vi "PassObserverSkill.vi"(8 "error in (no error)":errorcluster, 9 "Game in":refnum<class "Game.lvclass">, 10 "Robot":refnum<class "Robot.lvclass">, 11 "PassObserverSkill in":refnum<class "PassObserverSkill.lvclass">) -> (0 "error out":errorcluster, 1 "Boolean":bool, 2 "Robot":refnum<class "Robot.lvclass">, 3 "PassObserverSkill out":refnum<class "PassObserverSkill.lvclass">)   [LabVIEW 2018, in "PassObserverSkill.lvclass"]
uses:
  PassObserverSkill.lvclass
  Robot_class/Robot.lvclass
  Game_class/Game.lvclass
  Utilities_class/Utilities.lvclass
  Robot_class/roles.ctl
  Robot_class/tactics.ctl
  Object_class/Object.lvclass/Object.ctl
  Game_class/Game.lvclass/Game.ctl
  Team_class/Team.lvclass/Team.ctl
  Parameters_class/Parameters.lvclass/Parameters.ctl
  Robot_class/Robot.lvclass/Robot.ctl
  Game_class/Read OffensiveTeam.vi
  Game_class/Read FieldRef.vi
  Game_class/Read BallRef.vi
  Game_class/Read Parameters.lvclass.vi
  Parameters_class/Read AttakingOurselves.vi
  Object_class/Read x.vi
  Object_class/Read y.vi
  Team_class/Read RobotRef.vi
  Robot_class/Read tactic.vi
  Robot_class/Write dest_x.vi
  Robot_class/Write dest_y.vi
  Robot_class/Write dest_orientation.vi
  Ball_class/Ball.lvclass
  Ally_class/Ally.lvclass
  Field_class/Field.lvclass
  Parameters_class/Parameters.lvclass
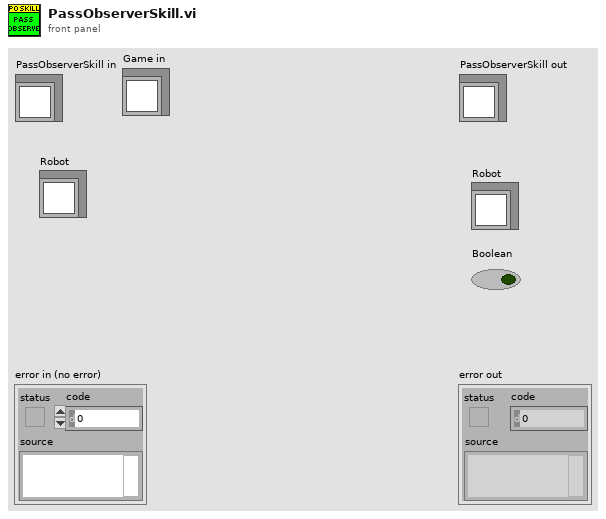
[diagram p1: front panel]
types:
  T1 = typedef "tactics.ctl" = enum16{"ReceivePassInFuturePoint", "Roller", "PrepareRollToPassRollerGoTo", "PrepareRollToPassReceiverGoTo", "WaitRoll", "PositionToRoll", "PenaltyAttacker", "PassObserver", "PenaltyDefense", "TableReceiverTactic", "Test", "DefendGoal", "Marker", "FollowAttacker", "DefendArea", "Shoot", "AttackerAimGoal", "AttackerBallOutOfField", "AttackerBlock", "AttackerStop", "Duelist", "Halt", "ZigZag", "GoTo", "Timeout", "KickToPassReceiver", "PositionToReceivePass", "WaitPass"}
  T2 = typedef "roles.ctl" = enum16{"Tabler", "TableFinalizer", "PrepareRollToPassRoller", "PrepareRollToPassReceiver", "SimplePassRoll", "SimplePassRollReceiver", "PenaltyDefense", "PreparePassReceiver 2", "PreparePassReceiver 1", "PassObserver", "Timeout", "Goto", "ZigZag", "None", "BallOutOfField", "DefenderArea", "Duelist", "AttackerStop", "FollowAttacker", "KeeperRole", "KickPenalty", "AttackerAimGoal", "AttackerBlock", "Marker", "Halt", "Shoot", "PassKicker", "PassReceiver", "TestRole", "PenaltyAttacker"}
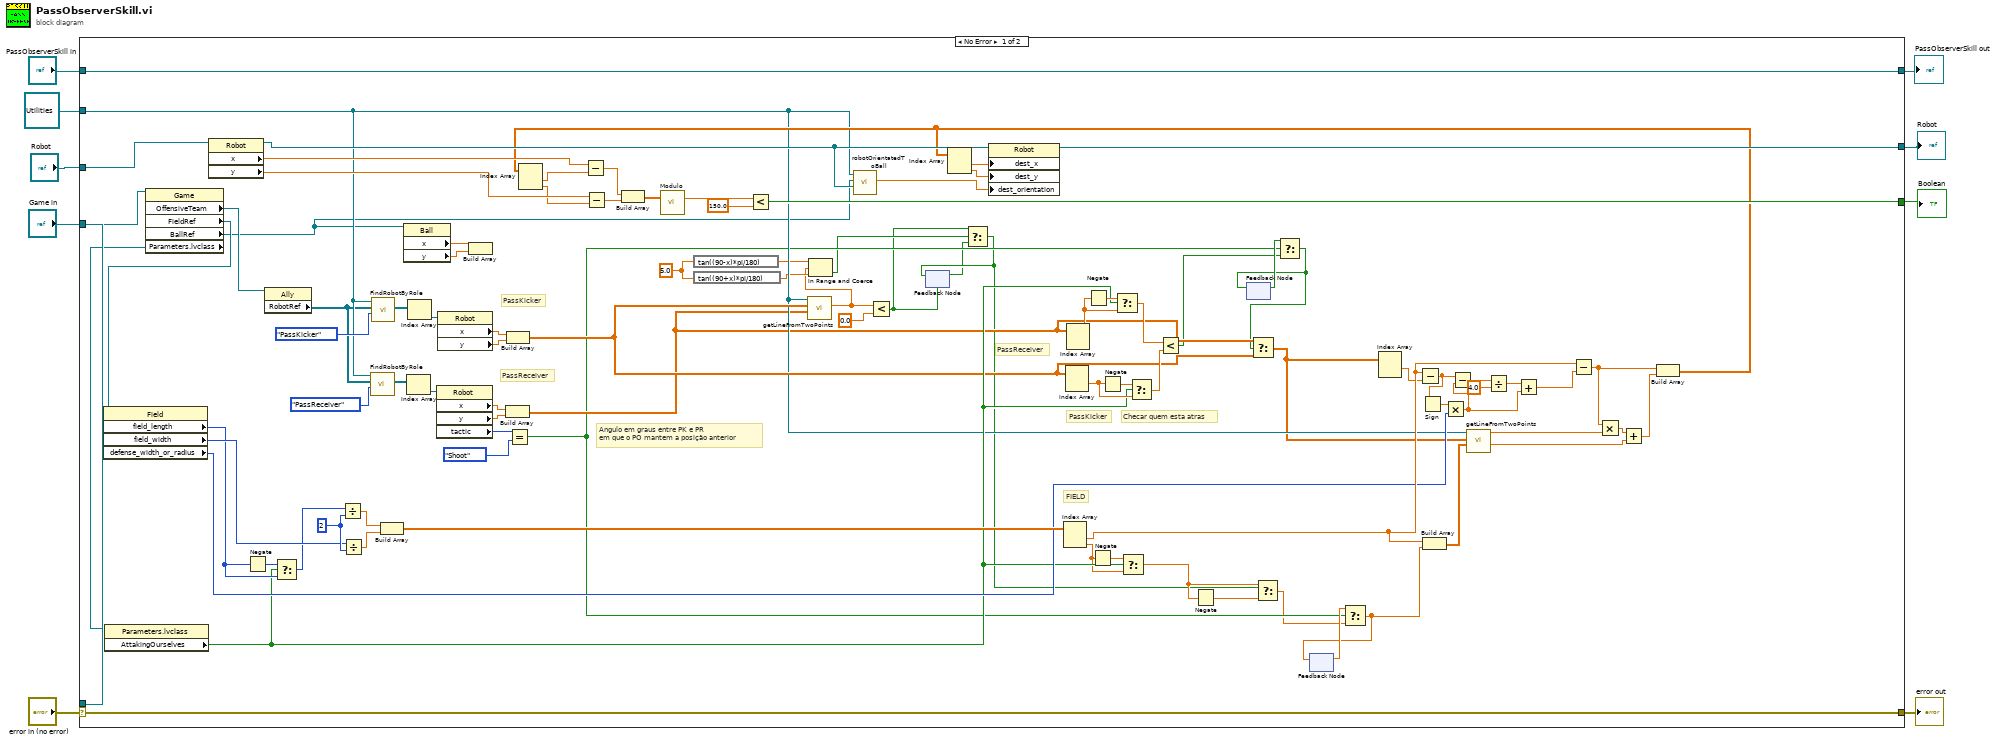
[diagram p0: block diagram]
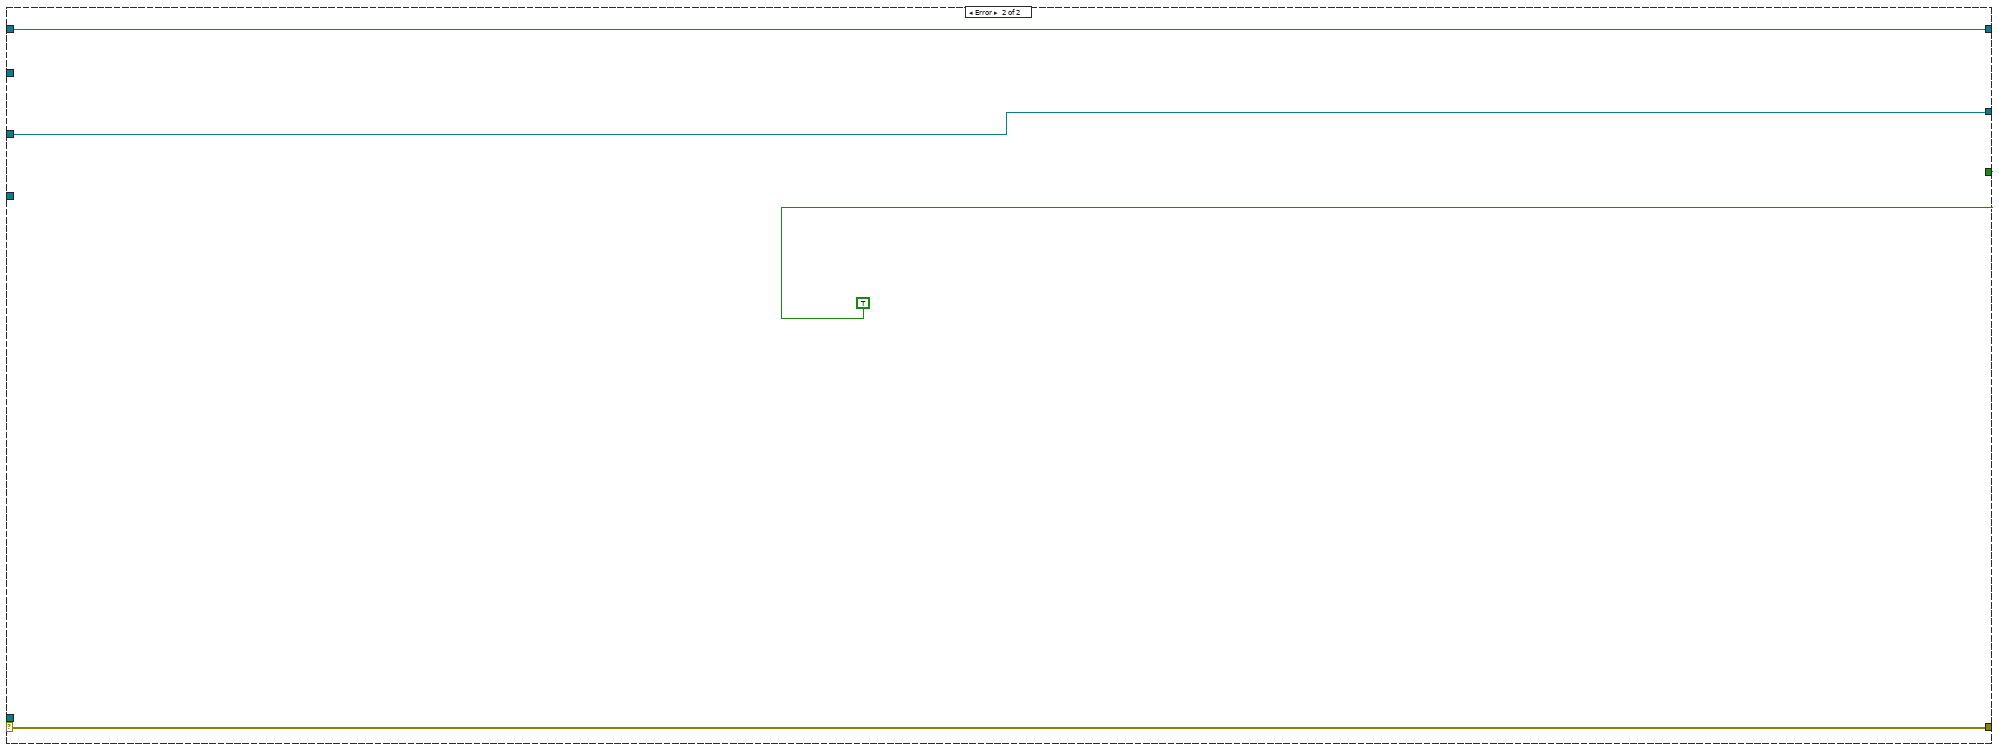
[diagram p2: hidden frame]
diagram:
  n1 = case shown="No Error" "error in (no error)" {
    selector: "error in (no error)" -> [w84 w107]
    tunnel: [w84 w107] -> w8
    tunnel: [w103 w106] -> w6
    tunnel: "PassObserverSkill in" -> [w103 w106]
    tunnel: "Robot" -> [w83 w105]
    tunnel: [w102 w105] -> w4
    tunnel: [w96 TRUE] -> w2
    tunnel: "Game in" -> [w95 _]
    tunnel: "Game in" -> [_ _]
    tunnel: refnum<class "Utilities.lvclass"> refnum ("Utilities in") -> [w31 _]
    frame No Error {
      w17 = 5.0
      w92 = 2
      # "Angulo em graus entre PK e PR \nem que o PO mantem a posição anterior"
      # "PassReceiver"
      # "Checar quem esta atras"
      # "PassReceiver"
      # "FIELD"
      # "PassKicker"
      # "PassKicker"
      n2 = property class="Game"(reference=w95) -> ("OffensiveTeam"=w94:refnum<class "Ally.lvclass">, "FieldRef"=w93:refnum<class "Field.lvclass">, "BallRef"=w10:refnum<class "Ball.lvclass">, "Parameters.lvclass"=w62:refnum<class "Parameters.lvclass">)  [unwired: 1 in, 2 out]
      n3 = property class="Field"(reference=w93) -> ("field_length"=w59:i32, "field_width"=w88:i32, "defense_width_or_radius"=w50:i32)  [unwired: 1 in, 2 out]
      n4 = property class="Parameters.lvclass"(reference=w62) -> ("AttakingOurselves"=w47:bool)  [unwired: 1 in, 2 out]
      n5 = property class="Robot"(reference=w83) -> (reference out=w85:refnum<class "Robot.lvclass">, "x"=w91:dbl, "y"=w90:dbl)  [unwired: 1 in, 1 out]
      n6 = Negate(x=w59) -> (-x=w60:i32)
      n7 = property class="Ally"(reference=w94) -> ("RobotRef"=w30:refnum<class "Robot.lvclass">[])  [unwired: 1 in, 2 out]
      n8 = Select(t=w60, s=w47, f=w59) -> (s? t:f=w58:i32)
      n9 = Divide(x=w58, y=w92) -> (x/y=w76:dbl)
      n10 = Divide(x=w88, y=w92) -> (x/y=w89:dbl)
      n11 = call "FindRobotByRole.vi"("role"=roles."PassReceiver" ("y"), "RobotRef"=w30, "Utilities in"=w31) -> ("Robots"=w35:refnum<class "Robot.lvclass">[])  [unwired: 6 in, 2 out]
      n12 = call "FindRobotByRole.vi"("role"=roles."PassKicker" ("y"), "RobotRef"=w30, "Utilities in"=w31) -> ("Robots"=w41:refnum<class "Robot.lvclass">[])  [unwired: 6 in, 2 out]
      n13 = Build Array(w76, w89) -> (w64:dbl[])
      n14 = property class="Ball"(reference=w10) -> ("x"=w78:dbl, "y"=w77:dbl)  [unwired: 1 in, 2 out]
      n15 = Index Array(array=w35) -> (element=w34:refnum<class "Robot.lvclass">)  [unwired: 1 in]
      n16 = Index Array(array=w41) -> (element=w40:refnum<class "Robot.lvclass">)  [unwired: 1 in]
      n17 = property class="Robot"(reference=w34) -> ("x"=w33:dbl, "y"=w32:dbl, "tactic"=w27:T1)  [unwired: 1 in, 2 out]
      n18 = property class="Robot"(reference=w40) -> ("x"=w39:dbl, "y"=w38:dbl)  [unwired: 1 in, 2 out]
      n19 = Build Array(w78, w77) -> ()  [unwired: 1 out]
      n20 = Build Array(w33, w32) -> (w29:dbl[])
      n21 = Build Array(w39, w38) -> (w37:dbl[])
      n22 = Equal?(x=w27, y=tactics."Shoot" ("tactic")) -> (x = y?=w24:bool)
      n23 = expression code="tan((90-x)*pi/180)"(w17) -> (w15:dbl)
      n24 = expression code="tan((90+x)*pi/180)"(w17) -> (w16:dbl)
      n25 = call "getLineFromTwoPoints.vi"("Point 2"=w29, "Point 1"=w37, "Utilities in"=w31) -> ("angular coef"=w14:dbl)  [unwired: 4 in, 4 out]
      n26 = In Range and Coerce(upper limit=w15, x=w14, lower limit=w16) -> (In Range?=w13:bool)  [unwired: 1 out]
      n27 = call "robotOrientatedToBall.vi"("Robot"=w85, "BallRef"=w10, "Utilities in"=w31) -> ("Orientation"=w86:dbl)  [unwired: 6 in, 2 out]
      n28 = Less?(x=w14, y=0.0) -> (x < y?=w12:bool)
      n29 = feedback #1(w12) -> (w11:bool)
      n30 = Select(t=w12, s=w13, f=w11) -> (s? t:f=w18:bool)
      n31 = feedback-in #1(w18) -> ()
      n32 = Index Array(array=w64) -> (element #1=w71:dbl, element #2=w44:dbl)  [unwired: 2 in]
      n33 = Index Array(array=w37) -> (element #1=w53:dbl)  [unwired: 2 in, 1 out]
      n34 = Index Array(array=w29) -> (element #1=w55:dbl)  [unwired: 2 in, 1 out]
      n35 = Negate(x=w55) -> (-x=w57:dbl)
      n36 = Negate(x=w44) -> (-x=w45:dbl)
      n37 = Negate(x=w53) -> (-x=w54:dbl)
      n38 = Select(t=w57, s=w47, f=w55) -> (s? t:f=w56:dbl)
      n39 = Select(t=w45, s=w47, f=w44) -> (s? t:f=w46:dbl)
      n40 = Select(t=w54, s=w47, f=w53) -> (s? t:f=w43:dbl)
      n41 = Less?(x=w56, y=w43) -> (x < y?=w20:bool)
      n42 = Negate(x=w46) -> (-x=w61:dbl)
      n43 = feedback #2() -> (w26:bool)  [unwired: 1 in]
      n44 = Select(t=w46, s=w18, f=w61) -> (s? t:f=w22:dbl)
      n45 = Select(t=w26, s=w24, f=w20) -> (s? t:f=w19:bool)
      n46 = feedback-in #2(w19) -> ()
      n47 = Select(t=w29, s=w19, f=w37) -> (s? t:f=w21:dbl[])
      n48 = feedback #3() -> (w25:dbl)  [unwired: 1 in]
      n49 = Select(t=w25, s=w24, f=w22) -> (s? t:f=w23:dbl)
      n50 = feedback-in #3(w23) -> ()
      n51 = Index Array(array=w21) -> (element #1=w65:dbl)  [unwired: 2 in, 1 out]
      n52 = Subtract(x=w71, y=w65) -> (x-y=w52:dbl)
      n53 = Sign(1:w52) -> (0:w51:dbl)
      n54 = Build Array(w71, w23) -> (w75:dbl[])
      n55 = Multiply(x=w51, y=w50) -> (x*y=w49:dbl)
      n56 = Subtract(x=w52, y=w49) -> (x-y=w74:dbl)
      n57 = call "getLineFromTwoPoints.vi"("Point 2"=w75, "Point 1"=w21, "Utilities in"=w31) -> ("linear coef"=w68:dbl, "angular coef"=w70:dbl)  [unwired: 4 in, 3 out]
      n58 = Divide(x=w74, y=4.0) -> (x/y=w72:dbl)
      n59 = Add(x=w72, y=w49) -> (x+y=w48:dbl)
      n60 = Subtract(x=w71, y=w48) -> (x-y=w67:dbl)
      n61 = Multiply(x=w67, y=w70) -> (x*y=w69:dbl)
      n62 = Add(x=w69, y=w68) -> (x+y=w66:dbl)
      n63 = Build Array(w67, w66) -> (w63:dbl[])
      n64 = Index Array(array=w63) -> (element #1=w80:dbl, element #2=w79:dbl)  [unwired: 2 in]
      n65 = Subtract(x=w91, y=w80) -> (x-y=w101:dbl)
      n66 = Subtract(x=w90, y=w79) -> (x-y=w100:dbl)
      n67 = Build Array(w101, w100) -> (w99:dbl[])
      n68 = call "Modulo.vi"("2D vector"=w99) -> ("Modulo"=w97:dbl)  [unwired: 10 in]
      n69 = Less?(x=w97, y=150.0) -> (x < y?=w96:bool)
      n70 = Index Array(array=w63) -> (element #1=w82:dbl, element #2=w81:dbl)  [unwired: 2 in]
      n71 = property class="Robot"(reference=w85, "dest_x"=w82, "dest_y"=w81, "dest_orientation"=w86) -> (reference out=w102:refnum<class "Robot.lvclass">)  [unwired: 1 in, 1 out]
    }
    frame Error {
    }
  }
  "error out" <- w8
  "PassObserverSkill out" <- w6
  "Robot" <- w4
  "Boolean" <- w2
